vi "GULP Out to data file.vi"() -> ()   [LabVIEW 2010]
uses:
  <vilib>/Utility/file.llb/Write To Spreadsheet File (string).vi
panel:
  in  "Path":path
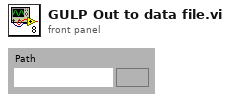
[diagram p1: front panel]
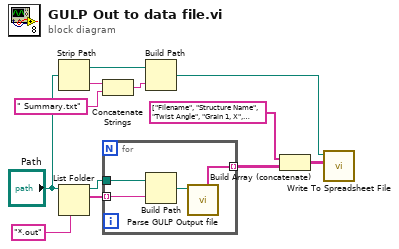
[diagram p0: block diagram]
diagram:
  n1 = Strip Path(path="Path") -> (stripped path=w1:path, name=w4:string)
  n2 = List Folder(path="Path", pattern="*.out") -> (path out=w12:path, filenames=w11:string[])  [unwired: 2 in, 2 out]
  n3 = Concatenate Strings(w4, " Summary.txt" ("string")) -> (w3:string)
  n4 = for {
    tunnel: w12 -> [w16]
    tunnel: w11 -> [w15] mode=indexing
    tunnel: [w13] -> w10 mode=indexing
    n5 = Build Path(base path=w16, name or relative path=w15) -> (appended path=w14:path)
    n6 = call "Parse GULP Output file.vi"("GULP output file"=w14) -> ("Data"=w13:string[])  [unwired: 5 in, 5 out]
  }
  n7 = Build Path(base path=w1, name or relative path=w3) -> (appended path=w6:path)
  n8 = Build Array (concatenate)(string[] ["Filename", "Structure Name", "Twist Angle", "Grain 1, X", "Grain 1, Y", "Grain 1, Z", "Grain 2, X", "Grain 2, Y", "Grain 2, Z", "Tilt Angle", "# of atoms", "|A|", "|B|", "|C|", "Total Lattice Energy (eV)", "Interfacial Energy (mJ/m²)"] ("Data 2"), w10) -> (w7:string[][])
  n9 = call-poly <vilib>:"Write To Spreadsheet File.vi"("2D data"=w7, "file path (dialog if empty)"=w6) -> ()  [unwired: 6 in, 1 out]
